vi "Calculation derivatives Batch.vi"(1 "Save path 2":path=path "F:/fh/传输D/2015谷粒实验/提取数据/原始总反射率/1-原始总反射率txt", 2 "Save path":path=path "F:/fh/传输D/2015谷粒实验/提取数据/原始总反射率/1-原始总反射率txt", 3 "file path (dialog if empty)":path=path "F:/fh/传输D/2015谷粒实验/提取数据/原始总反射率/1-原始总反射率txt") -> ()   [LabVIEW 2015]
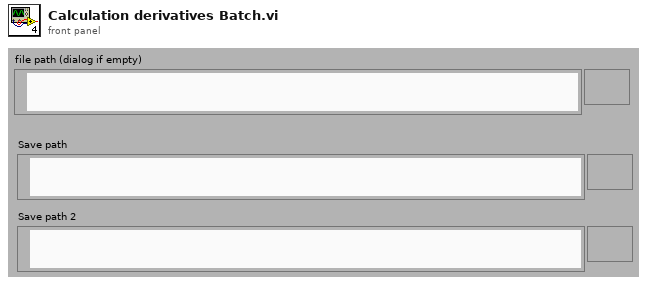
[diagram p1: front panel]
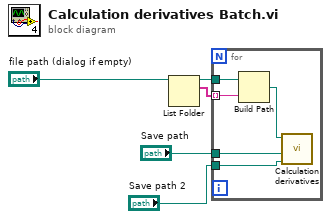
[diagram p0: block diagram]
diagram:
  n1 = List Folder(path="file path (dialog if empty)") -> (path out=w4:path, filenames=w3:string[])  [unwired: 1 in, 4 out]
  n2 = for {
    tunnel: w4 -> [w10]
    tunnel: w3 -> [w9] mode=indexing
    tunnel: "Save path" -> [w7]
    tunnel: "Save path 2" -> [w6]
    n3 = Build Path(base path=w10, name or relative path=w9) -> (appended path=w8:path)
    n4 = call "Calculation derivatives.vi"("Save path 2"=w6, "Save path"=w7, "file path (dialog if empty)"=w8) -> ()  [unwired: 9 in]
  }
